vi "Two Fgen Module.vi"() -> ()   [LabVIEW 2021]
uses:
  <instrlib>/niDigital/niDigital.llb/niDigital Selected Function.ctl
  <instrlib>/niDigital/niDigital.llb/niDigital Burst Pattern (Pass Fail).vi
panel:
  out "Sine Pass?":bool[](array[boolean])
  in  "Sine Wave":refnum<k15>="PXI1Slot2,PXI1Slot3" caption="resource name"
  out "Square Pass?":bool[](array[boolean])
  in  "Square Wave":refnum<k15>="PXI1Slot2,PXI1Slot3" caption="resource name"
  in  "I3C Generator Fgen Channel":string
  in  "I3C waveform":T1(ring)=enum."Noise"
  in  "I3C frequency":dbl=6.0
  in  "I3C amplitude":dbl=6.0
  in  "I3C Generator Fgen":refnum<k15>
  out "I3C Duration":dbl
  in  "duration":dbl
  out "I2C Duration":dbl
  in  "I2C Generator Fgen":refnum<k15>
  in  "I2C amplitude":dbl=6.0
  in  "I2C frequency":dbl=6.0
  in  "I2C waveform":T1(ring)=enum."Noise"
  in  "I2C Generator Fgen Channel":string
  out "error out":errorcluster
  in  "error in":errorcluster
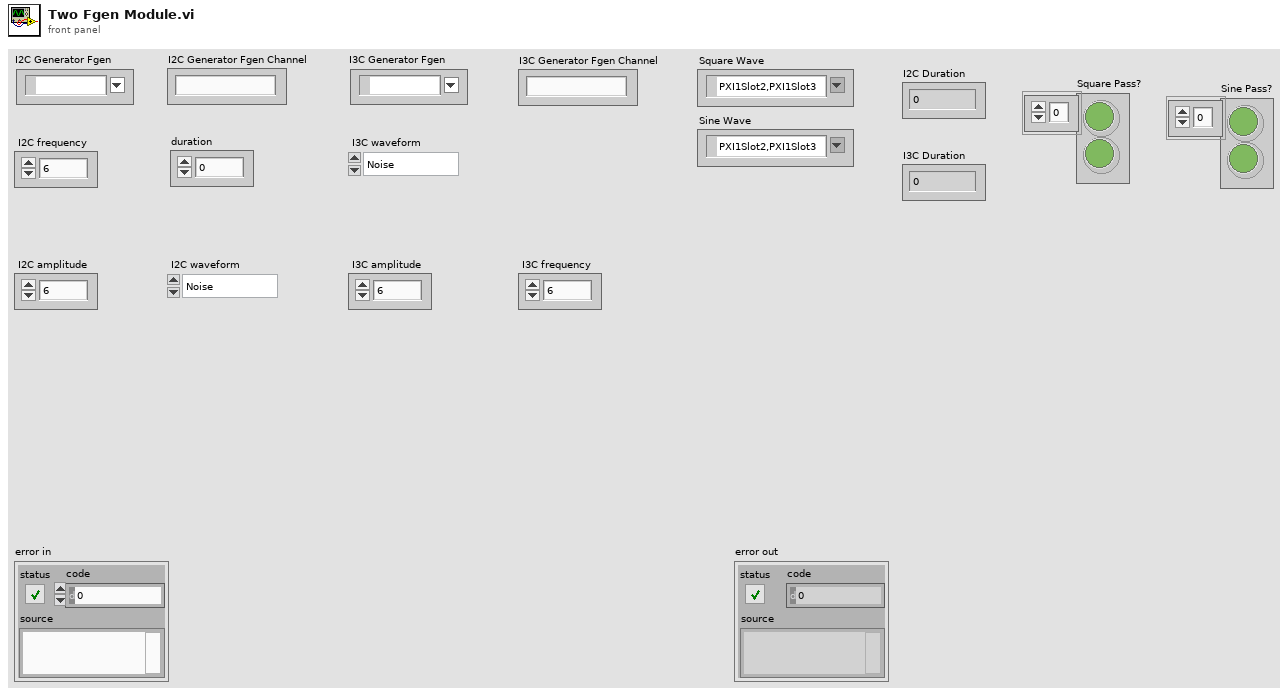
[diagram p1: front panel]
types:
  T1 = enum32{"Sine", "Square", "Triangle", "Ramp Up", "Ramp Down", "DC", "Noise", "User"}
  T2 = typedef "niDigital Selected Function.ctl" = i32
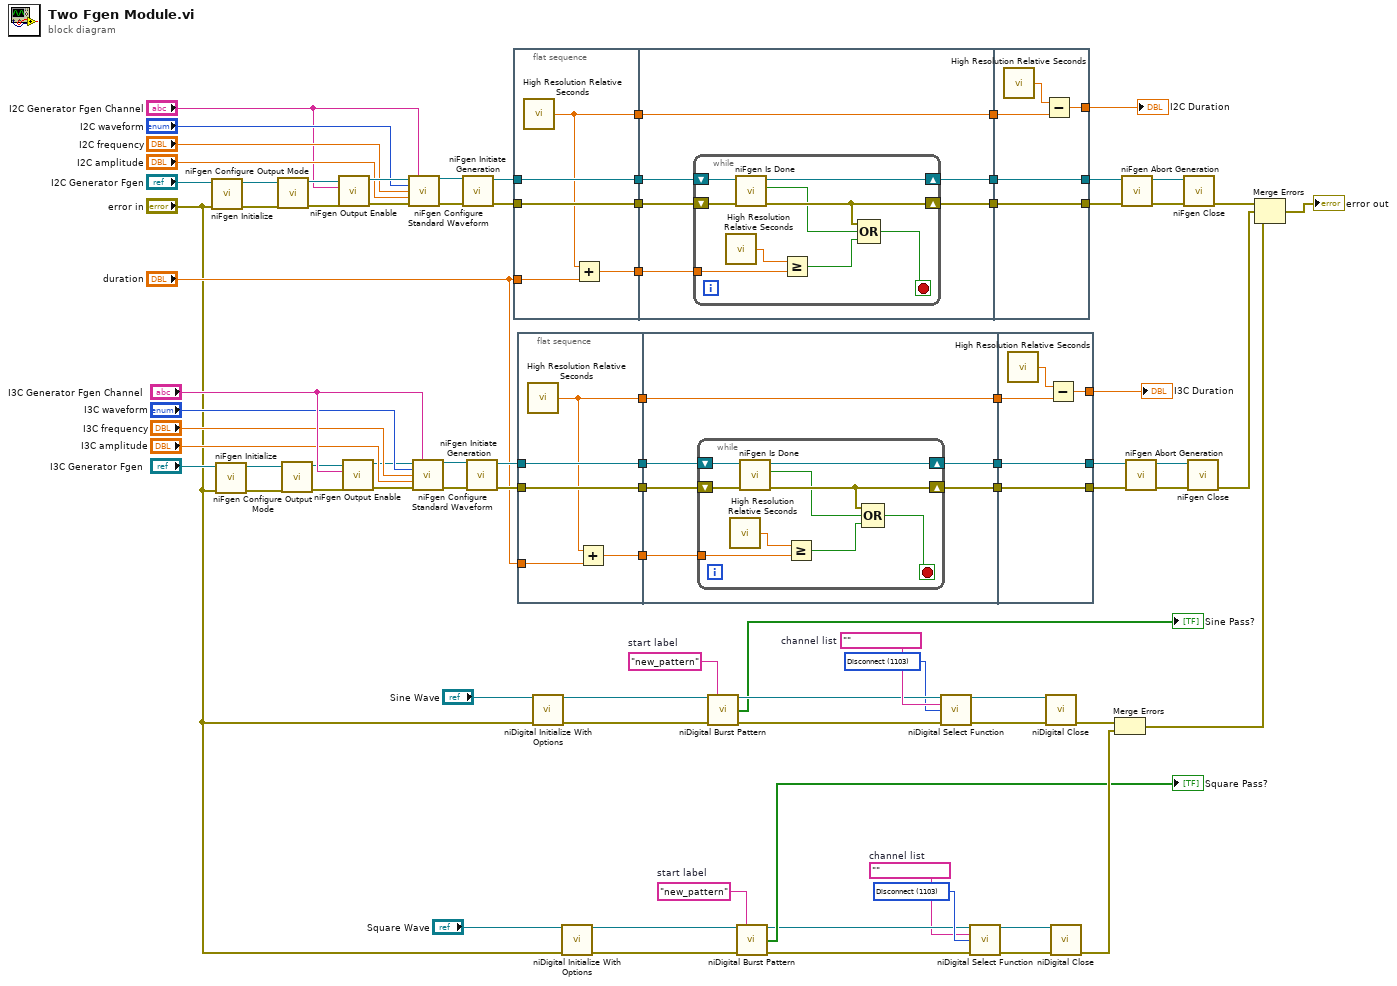
[diagram p0: block diagram]
diagram:
  w21 = T2 1103 items=["Digital"=1100, "PPMU"=1101, "Off"=1102, "Disconnect"=1103] ("function")
  w16 = ""  # channel list
  w25 = "new_pattern"  # start label
  w7 = T2 1103 items=["Digital"=1100, "PPMU"=1101, "Off"=1102, "Disconnect"=1103] ("function")
  w12 = ""  # channel list
  w3 = "new_pattern"  # start label
  n1 = call <instrlib>:"niFgen Initialize.vi"("error in (no error)"="error in", "Resource Name"="I2C Generator Fgen") -> ("error out"=w81:errorcluster, "Instrument Handle Out"=w84:refnum<k15>)  [unwired: 8 in]
  n2 = call <instrlib>:"niFgen Initialize.vi"("error in (no error)"="error in", "Resource Name"="I3C Generator Fgen") -> ("error out"=w33:errorcluster, "Instrument Handle Out"=w30:refnum<k15>)  [unwired: 8 in]
  n3 = call <instrlib>:"niFgen Configure Output Mode.vi"("error in (no error)"=w81, "Instrument Handle"=w84) -> ("error out"=w70:errorcluster, "Instrument Handle Out"=w80:refnum<k15>)  [unwired: 7 in]
  n4 = call <instrlib>:"niFgen Configure Output Mode.vi"("error in (no error)"=w33, "Instrument Handle"=w30) -> ("error out"=w43:errorcluster, "Instrument Handle Out"=w34:refnum<k15>)  [unwired: 7 in]
  n5 = call <instrlib>:"niFgen Output Enable.vi"("error in (no error)"=w70, "Channel Name"="I2C Generator Fgen Channel", "Instrument Handle"=w80) -> ("error out"=w82:errorcluster, "Instrument Handle Out"=w79:refnum<k15>)  [unwired: 7 in]
  n6 = call <instrlib>:"niFgen Output Enable.vi"("error in (no error)"=w43, "Channel Name"="I3C Generator Fgen Channel", "Instrument Handle"=w34) -> ("error out"=w32:errorcluster, "Instrument Handle Out"=w35:refnum<k15>)  [unwired: 7 in]
  n7 = call <instrlib>:"niFgen Configure Standard Waveform.vi"("Instrument Handle"=w79, "Channel Name"="I2C Generator Fgen Channel", "Waveform"="I2C waveform", "Frequency"="I2C frequency", "Amplitude"="I2C amplitude", "error in (no error)"=w82) -> ("Instrument Handle Out"=w78:refnum<k15>, "error out"=w83:errorcluster)  [unwired: 8 in]
  n8 = call <instrlib>:"niFgen Configure Standard Waveform.vi"("Instrument Handle"=w35, "Channel Name"="I3C Generator Fgen Channel", "Waveform"="I3C waveform", "Frequency"="I3C frequency", "Amplitude"="I3C amplitude", "error in (no error)"=w32) -> ("Instrument Handle Out"=w36:refnum<k15>, "error out"=w31:errorcluster)  [unwired: 8 in]
  n9 = call <instrlib>:"niFgen Initiate Generation.vi"("error in (no error)"=w83, "Instrument Handle"=w78) -> ("error out"=w75:errorcluster, "Instrument Handle Out"=w77:refnum<k15>)  [unwired: 8 in]
  n10 = call <instrlib>:"niFgen Initiate Generation.vi"("error in (no error)"=w31, "Instrument Handle"=w36) -> ("error out"=w39:errorcluster, "Instrument Handle Out"=w37:refnum<k15>)  [unwired: 8 in]
  n11 = flat-sequence {
    tunnel: w75 -> [w88]
    tunnel: w77 -> [w89]
    tunnel: [w89] -> w64
    tunnel: [w88] -> w63
    tunnel: [w87] -> w59
    tunnel: "duration" -> [w86]
    tunnel: [w85] -> w57
    tunnel: w64 -> [w95]
    tunnel: w63 -> [w93]
    tunnel: [w94] -> w62
    tunnel: [w92] -> w61
    tunnel: [w91] -> w60
    tunnel: w59 -> [w91]
    tunnel: w57 -> [w90]
    tunnel: [w108] -> w74
    tunnel: [w109] -> w76
    tunnel: w62 -> [w109]
    tunnel: w61 -> [w108]
    tunnel: w60 -> [w106]
    tunnel: [w105] -> w58
    frame #0 {
      n12 = call <vilib>:"High Resolution Relative Seconds.vi"() -> ("relative seconds"=w87:dbl)
      n13 = Add(x=w87, y=w86) -> (x+y=w85:dbl)
    }
    frame #1 {
      n14 = while {
        shift-right: [w103] -> w94
        shift-left: w95 -> [w104]
        shift-right: [w101] -> w92
        shift-left: w93 -> [w102]
        tunnel: w90 -> [w98]
        stop <- w100 stop-if-true
        n15 = call <vilib>:"High Resolution Relative Seconds.vi"() -> ("relative seconds"=w99:dbl)
        n16 = call <instrlib>:"niFgen Is Done.vi"("error in (no error)"=w102, "Instrument Handle"=w104) -> ("error out"=w101:errorcluster, "Done"=w96:bool, "Instrument Handle Out"=w103:refnum<k15>)  [unwired: 7 in]
        n17 = Greater Or Equal?(x=w99, y=w98) -> (x >= y?=w97:bool)
        n18 = Compound Arithmetic op=OR(w101, w96, w97) -> (w100:bool)
      }
    }
    frame #2 {
      n19 = call <vilib>:"High Resolution Relative Seconds.vi"() -> ("relative seconds"=w107:dbl)
      n20 = Subtract(x=w107, y=w106) -> (x-y=w105:dbl)
    }
  }
  n21 = flat-sequence {
    tunnel: w39 -> [w113]
    tunnel: w37 -> [w114]
    tunnel: [w114] -> w56
    tunnel: [w113] -> w55
    tunnel: [w112] -> w54
    tunnel: "duration" -> [w111]
    tunnel: [w110] -> w53
    tunnel: w56 -> [w120]
    tunnel: w55 -> [w118]
    tunnel: [w119] -> w52
    tunnel: [w117] -> w51
    tunnel: [w116] -> w50
    tunnel: w54 -> [w116]
    tunnel: w53 -> [w115]
    tunnel: [w133] -> w40
    tunnel: [w134] -> w38
    tunnel: w52 -> [w134]
    tunnel: w51 -> [w133]
    tunnel: w50 -> [w131]
    tunnel: [w130] -> w49
    frame #0 {
      n22 = call <vilib>:"High Resolution Relative Seconds.vi"() -> ("relative seconds"=w112:dbl)
      n23 = Add(x=w112, y=w111) -> (x+y=w110:dbl)
    }
    frame #1 {
      n24 = while {
        shift-right: [w128] -> w119
        shift-left: w120 -> [w129]
        shift-right: [w126] -> w117
        shift-left: w118 -> [w127]
        tunnel: w115 -> [w123]
        stop <- w125 stop-if-true
        n25 = call <vilib>:"High Resolution Relative Seconds.vi"() -> ("relative seconds"=w124:dbl)
        n26 = call <instrlib>:"niFgen Is Done.vi"("error in (no error)"=w127, "Instrument Handle"=w129) -> ("error out"=w126:errorcluster, "Done"=w121:bool, "Instrument Handle Out"=w128:refnum<k15>)  [unwired: 7 in]
        n27 = Greater Or Equal?(x=w124, y=w123) -> (x >= y?=w122:bool)
        n28 = Compound Arithmetic op=OR(w126, w121, w122) -> (w125:bool)
      }
    }
    frame #2 {
      n29 = call <vilib>:"High Resolution Relative Seconds.vi"() -> ("relative seconds"=w132:dbl)
      n30 = Subtract(x=w132, y=w131) -> (x-y=w130:dbl)
    }
  }
  n31 = call <instrlib>:"niDigital Initialize With Options.vi"("resource name"="Sine Wave", "error in"="error in") -> ("instrument handle"=w4:refnum<k15>, "error out"=w5:errorcluster)  [unwired: 12 in]
  n32 = call <instrlib>:"niDigital Initialize With Options.vi"("resource name"="Square Wave", "error in"="error in") -> ("instrument handle"=w24:refnum<k15>, "error out"=w23:errorcluster)  [unwired: 12 in]
  n33 = call-poly <instrlib>:"niDigital Burst Pattern.vi"("instrument handle"=w4, "start label"=w3, "error in"=w5) -> ("instrument handle out"=w8:refnum<k15>, "pass"=→"Sine Pass?":bool[], "error out"=w9:errorcluster)  [unwired: 10 in]
  n34 = call-poly <instrlib>:"niDigital Burst Pattern.vi"("instrument handle"=w24, "start label"=w25, "error in"=w23) -> ("instrument handle out"=w20:refnum<k15>, "pass"=→"Square Pass?":bool[], "error out"=w19:errorcluster)  [unwired: 10 in]
  n35 = call <instrlib>:"niDigital Select Function.vi"("instrument handle"=w8, "channel list"=w12, "function"=w7, "error in"=w9) -> ("instrument handle out"=w10:refnum<k15>, "error out"=w11:errorcluster)  [unwired: 10 in]
  n36 = call <instrlib>:"niDigital Select Function.vi"("instrument handle"=w20, "channel list"=w16, "function"=w21, "error in"=w19) -> ("instrument handle out"=w18:refnum<k15>, "error out"=w17:errorcluster)  [unwired: 10 in]
  n37 = call <instrlib>:"niDigital Close.vi"("instrument handle"=w10, "error in"=w11) -> ("error out"=w14:errorcluster)  [unwired: 13 in]
  n38 = call <instrlib>:"niDigital Close.vi"("instrument handle"=w18, "error in"=w17) -> ("error out"=w26:errorcluster)  [unwired: 13 in]
  n39 = Merge Errors(w14, w26) -> (w2:errorcluster)
  n40 = call <instrlib>:"niFgen Abort Generation.vi"("error in (no error)"=w74, "Instrument Handle"=w76) -> ("error out"=w72:errorcluster, "Instrument Handle Out"=w73:refnum<k15>)  [unwired: 8 in]
  n41 = call <instrlib>:"niFgen Abort Generation.vi"("error in (no error)"=w40, "Instrument Handle"=w38) -> ("error out"=w42:errorcluster, "Instrument Handle Out"=w41:refnum<k15>)  [unwired: 8 in]
  n42 = call <instrlib>:"niFgen Close.vi"("error in (no error)"=w72, "Instrument Handle"=w73) -> ("error out"=w71:errorcluster)  [unwired: 9 in]
  n43 = call <instrlib>:"niFgen Close.vi"("error in (no error)"=w42, "Instrument Handle"=w41) -> ("error out"=w27:errorcluster)  [unwired: 9 in]
  n44 = Merge Errors(w71, w27, w2) -> (→"error out":errorcluster)
  "I2C Duration" <- w58
  "I3C Duration" <- w49
